vi "Toggle Power.vi"(8 "error in (no error)":errorcluster, 10 "Power On?":bool, 11 "Vacuum Pumps in":refnum<class "Vacuum Pumps.lvclass">) -> (0 "error out":errorcluster, 3 "Vacuum Pumps out":refnum<class "Vacuum Pumps.lvclass">)   [LabVIEW 2021, in "Vacuum Pumps.lvclass"]
uses:
  Vacuum Pumps.lvclass
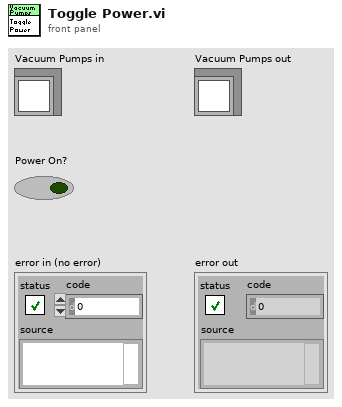
[diagram p1: front panel]
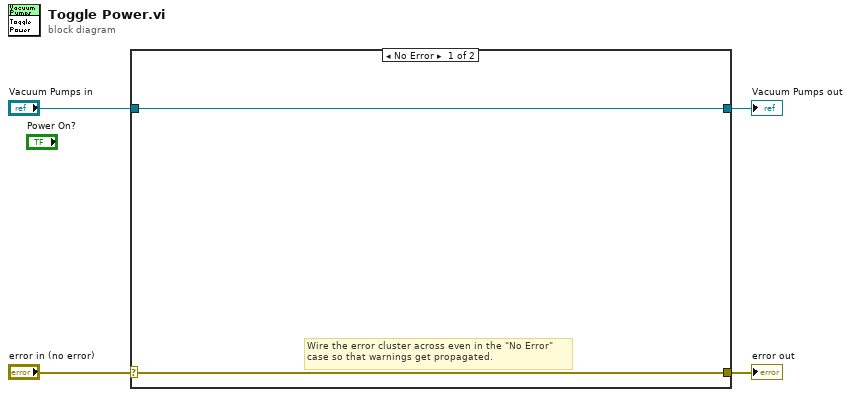
[diagram p0: block diagram]
diagram:
  n1 = case shown="No Error" "error in (no error)" {
    selector: "error in (no error)" -> [w5 w8]
    tunnel: [w5 w8] -> w3
    tunnel: [w6 w7] -> w1
    tunnel: "Vacuum Pumps in" -> [w6 w7]
    frame No Error {
      # "Wire the error cluster across even in the \"No Error\"\ncase so that warnings get propagated."
    }
    frame Error {
    }
  }
  "error out" <- w3
  "Vacuum Pumps out" <- w1
